vi "Filter Tree Item Open Event.vi"(8 "error in (no error)":errorcluster, 10 "TreeItemOpenMsg":refnum<class "TreeItemOpenMsg.lvclass">, 11 "IEventFilter in":refnum<class "IEventFilter.lvclass">) -> (0 "error out":errorcluster, 1 "Discard?":bool, 3 "IEventFilter out":refnum<class "IEventFilter.lvclass">)   [LabVIEW 2018, in "MVA Framework.lvlib" / "ActorEvents.lvlib" / "IEventFilter.lvclass"]
doc: "过滤树形项打开事件"
uses:
  IEventFilter.lvclass
  IEventAggregator Messages/TreeItemOpenMsg/TreeItemOpenMsg.lvclass
panel:
  # "No additional\nEvent Data"
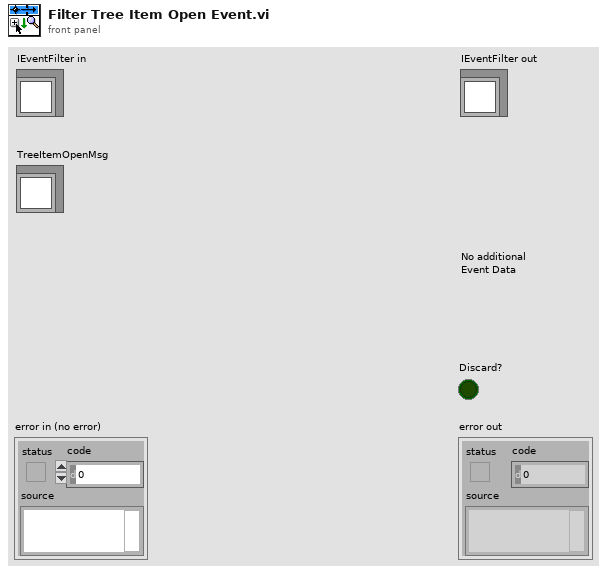
[diagram p1: front panel]
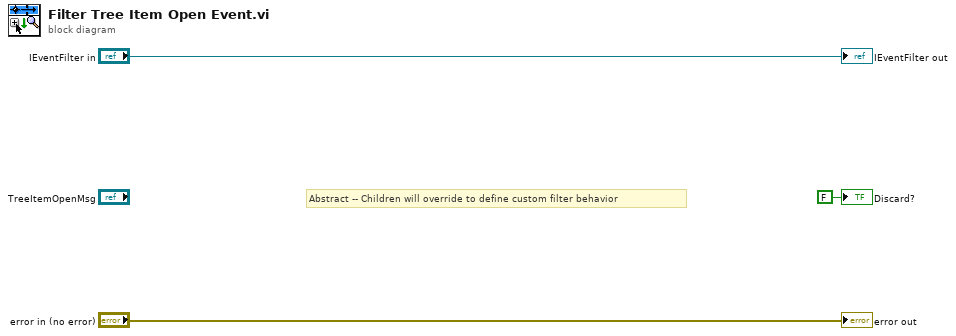
[diagram p0: block diagram]
diagram:
  # "Abstract -- Children will override to define custom filter behavior"
  "error out" <- "error in (no error)"
  "IEventFilter out" <- "IEventFilter in"
  "Discard?" <- FALSE ("Discard?")
